vi "PGPASS.Write.vi"(8 "error in":errorcluster, 11 "Connections":T1[](array[typedef])) -> (0 "error out":errorcluster)   [LabVIEW 2019, in "PGPASS.lvlib"]
uses:
  PGPASS.lvlib
  PGPASS.Connection Information.ctl
  <vilib>/IgorTitov/AES/Advanced Encryption Standard (AES).lvlib
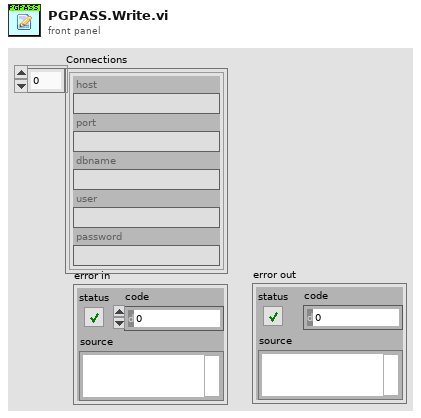
[diagram p1: front panel]
types:
  T1 = typedef "PGPASS.lvlib/PGPASS.Connection Information.ctl" = cluster{"host":string, "port":string, "dbname":string, "user":string, "password":string}
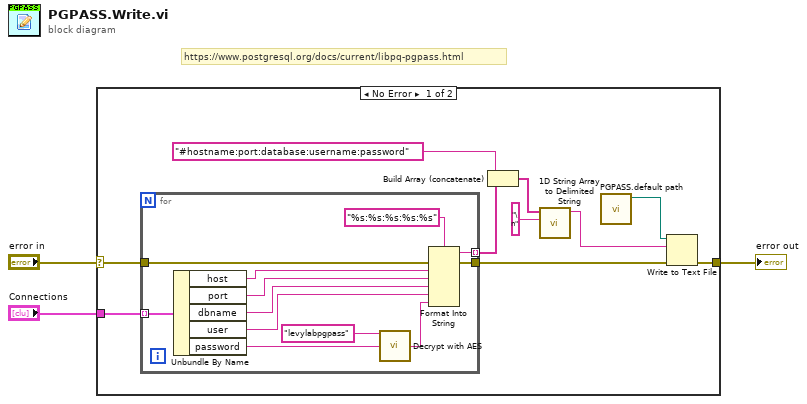
[diagram p0: block diagram]
diagram:
  # "https://www.postgresql.org/docs/current/libpq-pgpass.html"
  n1 = case shown="No Error" "error in" {
    selector: "error in" -> [w9 w26]
    tunnel: [w12 w26] -> w3
    tunnel: "Connections" -> [w13 _]
    frame No Error {
      n2 = for {
        tunnel: [w24] -> w7 mode=indexing
        tunnel: w13 -> [w23] mode=indexing
        tunnel: [w20] -> w11
        tunnel: w9 -> [w18]
        n3 = Unbundle By Name(w23) -> ("host"=w16:string, "port"=w19:string, "dbname"=w21:string, "user"=w22:string, "password"=w17:string)
        n4 = call <vilib>:"Decrypt with AES.vi"("Password.In"="levylabpgpass", "Encrypted Text In"=w17) -> ("Decrypted Text Out"=w14:string)  [unwired: 12 in, 1 out]
        n5 = Format Into String(format string="%s:%s:%s:%s:%s", error in=w18, w16, w19, w21, w22, w14) -> (resulting string=w24:string, error out=w20:errorcluster)  [unwired: 1 in]
      }
      n6 = Build Array (concatenate)("#hostname:port:database:username:password" ("format string"), w7) -> (w6:string[])
      n7 = call <vilib>:"1D String Array to Delimited String.vi"("delimiter"="\n", "string array"=w6) -> ("delimited string"=w5:string)  [unwired: 9 in]
      n8 = call "PGPASS.default path.vi"() -> ("PGPASS path"=w10:path)  [unwired: 10 in, 1 out]
      n9 = Write to Text File(file (use dialog)=w10, text=w5, error in=w11) -> (error out=w12:errorcluster)  [unwired: 1 in, 2 out]
    }
    frame Error {
    }
  }
  "error out" <- w3
